vi "U2000_USB_PM_Configure_Correction.vi"(8 "error in (no error)":errorcluster, 10 "Frequency (5E+7 Hz)":dbl=50000000.0, 11 "VISA resource name":refnum<visa-resource-name>) -> (0 "error out":errorcluster, 3 "VISA resource name out":refnum<visa-resource-name>)   [LabVIEW 2015]
doc: "Sets the correction frequency."
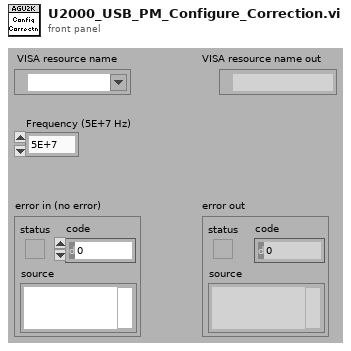
[diagram p1: front panel]
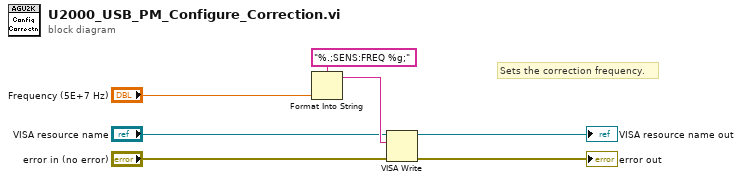
[diagram p0: block diagram]
diagram:
  # "Sets the correction frequency."
  n1 = Format Into String(format string="%.;SENS:FREQ %g;", "Frequency (5E+7 Hz)") -> (resulting string=w5:string)  [unwired: 2 in, 1 out]
  n2 = VISA Write(VISA resource name="VISA resource name", write buffer=w5, error in (no error)="error in (no error)") -> (VISA resource name out=→"VISA resource name out":refnum<visa-resource-name>, error out=→"error out":errorcluster)  [unwired: 1 out]
